vi "Cross_wire_stats.vi"(0 "Eng Units":dbl[][](array[numeric]) format="%.2f", 2 "Info Index":i32, 5 "Indicies":i32[](array[numeric]), 9 "Inst names":string[](array[string]), 11 "Shift in":dbl[](array[numeric]) format="%.2f", 12 "Block No":i32) -> (4 "Results file string array":string[](array[string]), 15 "Shift out":dbl[](array[numeric]) format="%.2f")   [LabVIEW 2010]
uses:
  Globals/Meas_global.vi
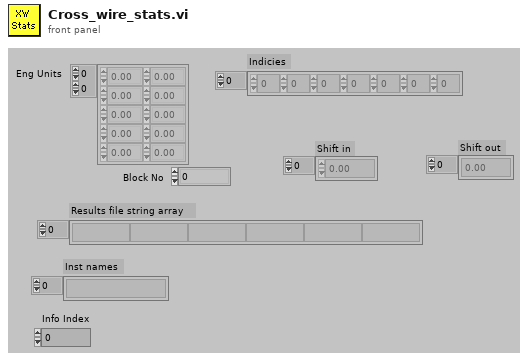
[diagram p1: front panel]
types:
  T1 = typedef "Velocity_cluster.ctl" = cluster{"Name":string, "U":dbl, "u^2":dbl, "u^3/(u^2)^(1.5)":dbl, "u^4/(u^2)^2 -3":dbl, "% u'/U":dbl, "Mean % Err":dbl, "u^4":dbl}
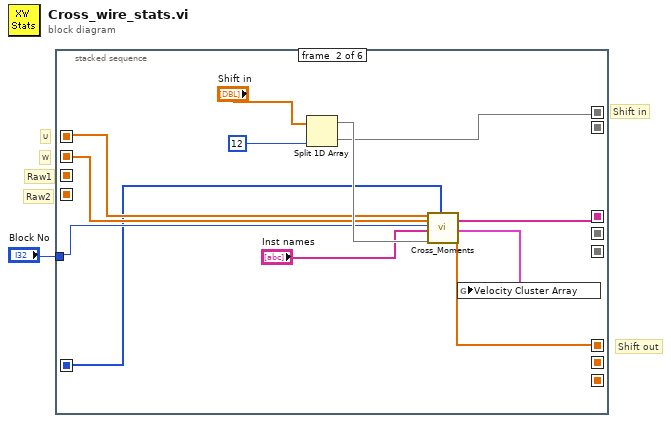
[diagram p0: block diagram]
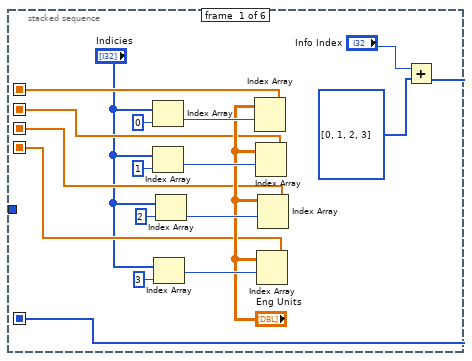
[diagram p2: hidden frame]
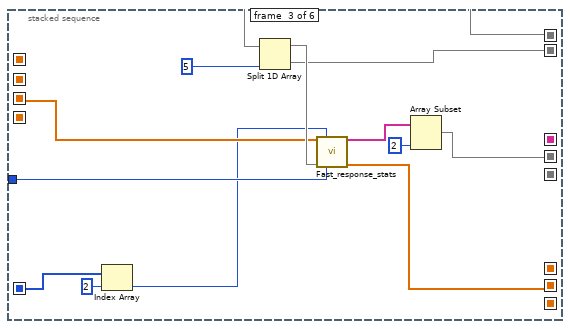
[diagram p3: hidden frame]
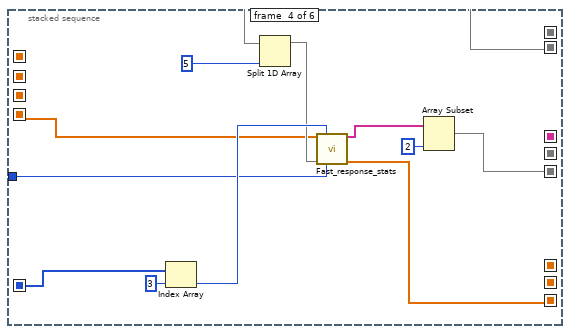
[diagram p4: hidden frame]
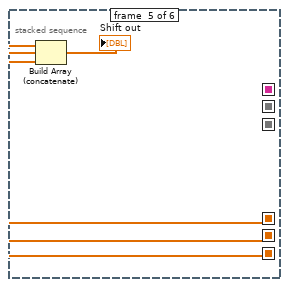
[diagram p5: hidden frame]
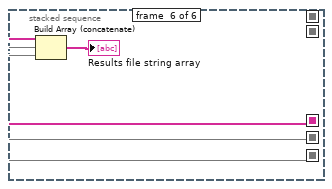
[diagram p6: hidden frame]
diagram:
  # "Shift out"
  # "Shift in"
  # "Raw2"
  # "Raw1"
  # "W"
  # "U"
  n1 = stacked-sequence {
    seq-local: [w9 _ _ _ _ _] -> [_ w26 _ _ _ _]
    seq-local: [w8 _ _ _ _ _] -> [_ w25 _ _ _ _]
    seq-local: [w7 _ _ _ _ _] -> [_ _ w35 _ _ _]
    seq-local: [w6 _ _ _ _ _] -> [_ _ _ w47 _ _]
    seq-local: [w3 _ _ _ _ _] -> [_ w20 w42 w54 _ _]
    seq-local: [_ w28 _ _ _ _] -> [_ _ w38 _ _ _]
    seq-local: [_ w27 _ _ _ _] -> [_ _ _ _ w59 _]
    seq-local: [_ w22 _ _ _ _] -> [_ _ _ _ _ w63]
    seq-local: [_ _ w31 _ _ _] -> [_ _ _ _ _ w62]
    seq-local: [_ _ _ w44 _ _] -> [_ _ _ _ _ w61]
    seq-local: [_ _ w36 _ _ _] -> [_ _ _ _ w58 _]
    seq-local: [_ _ _ w48 _ _] -> [_ _ _ _ w57 _]
    seq-local: [_ _ w37 _ _ _] -> [_ _ _ w49 _ _]
    tunnel: "Block No" -> [_ w24 w40 w51 _ _]
    frame #0 {
      n2 = Index Array(array="Indicies", index=0) -> (element=w14:i32)
      n3 = Index Array(array="Indicies", index=1) -> (element=w13:i32)
      n4 = Index Array(array="Indicies", index=3) -> (element=w11:i32)
      n5 = Index Array(array="Indicies", index=2) -> (element=w12:i32)
      n6 = Index Array(array="Eng Units", index (row)=w14) -> (element=w9:dbl[])  [unwired: 1 in]
      n7 = Index Array(array="Eng Units", index (row)=w13) -> (element=w8:dbl[])  [unwired: 1 in]
      n8 = Index Array(array="Eng Units", index (row)=w11) -> (element=w6:dbl[])  [unwired: 1 in]
      n9 = Index Array(array="Eng Units", index (row)=w12) -> (element=w7:dbl[])  [unwired: 1 in]
      n10 = Add(x="Info Index", y=i32[] [0, 1, 2, 3] ("x+y")) -> (x+y=w3:i32[])
    }
    frame #1 {
      n11 = Split 1D Array(array="Shift in", index=12) -> (first subarray=w29:dbl[], second subarray=w28:dbl[])
      n12 = call "Cross_Moments.vi"("U"=w26, "W"=w25, "Block No"=w24, "Inst names"="Inst names", "Shift in"=w29, "Indicies"=w20) -> ("All Results for file"=w22:string[], "Velocity Cluster Array Out"=w19:T1[], "Shift out"=w27:dbl[])  [unwired: 3 in, 8 out]
      n13 = global write "Meas_global.vi" "Velocity Cluster Array"(w19) -> ()
    }
    frame #2 {
      n14 = Index Array(array=w42, index=2) -> (element=w34:i32)
      n15 = Split 1D Array(array=w38, index=5) -> (first subarray=w39:dbl[], second subarray=w37:dbl[])
      n16 = call "Fast_response_stats.vi"("U"=w35, "Index"=w34, "Shift in"=w39, "Block No"=w40) -> ("Results file string array"=w33:string[], "Shift out"=w36:dbl[])  [unwired: 10 out]
      n17 = Array Subset(array=w33, length=2) -> (w31:string[])  [unwired: 1 in]
    }
    frame #3 {
      n18 = Index Array(array=w54, index=3) -> (element=w52:i32)
      n19 = Split 1D Array(array=w49, index=5) -> (first subarray=w50:dbl[])  [unwired: 1 out]
      n20 = call "Fast_response_stats.vi"("U"=w47, "Index"=w52, "Shift in"=w50, "Block No"=w51) -> ("Results file string array"=w45:string[], "Shift out"=w48:dbl[])  [unwired: 10 out]
      n21 = Array Subset(array=w45, length=2) -> (w44:string[])  [unwired: 1 in]
    }
    frame #4 {
      n22 = Build Array (concatenate)(w59, w58, w57) -> (→"Shift out":dbl[])
    }
    frame #5 {
      n23 = Build Array (concatenate)(w63, w62, w61) -> (→"Results file string array":string[])
    }
  }
